vi "DictVectorizer.vi"(8 "error in":errorcluster caption="entrée d'erreur", 11 "DictVectorizer":T1={"dtype"="float", "separator"="=", "sparse"=TRUE, "sort"=TRUE}) -> (0 "error out":errorcluster caption="sortie d'erreur", 3 "DictVectorizer.lvclass":refnum<class "DictVectorizer.lvclass">)   [LabVIEW 2020]
doc: "Transforms lists of feature-value mappings to vectors.\n\nThis transformer turns lists of mappings (dict-like objects) of feature names to feature values into Numpy arrays or scipy.sparse matrices for use with scikit-learn estimators.\n\nWhen feature values are strings, this transformer will do a binary one-hot (aka one-of-K) coding: one boolean-valued feature is constructed for each of the possible string values that the feature can take on. For instance, a feature “f” that can take on the values “ham” and “spam” will become two features in the output, one signifying “f=ham”, the other “f=spam”.\n\nHowever, note that this transformer will only do a binary one-hot encoding when feature values are of type string. If categorical features are represented as numeric values such as int, the DictVectorizer can be followed by sklearn.preprocessing.OneHotEncoder to complete binary one-hot encoding.\n\nFeatures that do not occur in a sample (mapping) will have a zero value in the resulting array/matrix.\n\n\nParameters : \n\n- dtyped : type, default=np.float64\nThe type of feature values. Passed to Numpy array/scipy.sparse matrix constructors as the dtype argument.\n\n- separator : str, default=”=”\nSeparator string used when constructing new features for one-hot coding.\n\n- sparse : bool, default=True\nWhether transform should produce scipy.sparse matrices.\n\n- sort : bool, default=True\nWhether feature_names_ and vocabulary_ should be sorted when fitting.\n\n\nMethods : \n\n- Fit : Learn a list of feature name -> indices mappings.\n\nParameters : X : Mapping or iterable over Mappings\n Dict(s) or Mapping(s) from feature names (arbitrary Python objects) to feature values (strings or convertible to dtype).\n\n- Fit Transform : Learn a list of feature name -> indices mappings and transform X. Like fit(X) followed by transform(X), but does not require materializing X in memory.\n\nParameters : X : Mapping or iterable over Mappings\n Dict(s) or Mapping(s) from feature names (arbitrary Python objects) to feature values (strings or convertible to dtype).\n\nReturns : Xa : {array, sparse matrix}\n Feature vectors; always 2-d.\n \n- Get Feature Names : Returns a list of feature names, ordered by their indices. If one-of-K coding is applied to categorical features, this will include the constructed feature names but not the original ones.\n\n\n- Transform : Transform feature->value dicts to array or sparse matrix. Named features not encountered during fit or fit_transform will be silently ignored.\n\nParameters : X : Mapping or iterable over Mappings of shape (n_samples,)\n Dict(s) or Mapping(s) from feature names (arbitrary Python objects) to feature values (strings or convertible to dtype).\n\nReturns : Xa : {array, sparse matrix}\n Feature vectors; always 2-d."
uses:
  DictVectorizer.lvclass
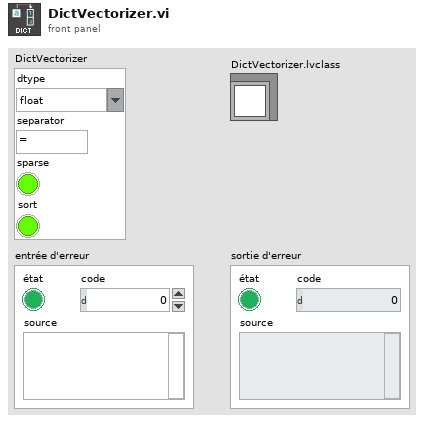
[diagram p1: front panel]
types:
  T1 = cluster{"dtype":string, "separator":string, "sparse":bool, "sort":bool}
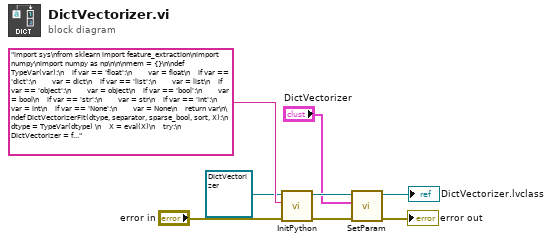
[diagram p0: block diagram]
diagram:
  n1 = call-dynamic "InitPython.vi"("error in (no error)"="error in", "Python Instruction"="import sys\nfrom sklearn import feature_extraction\nimport numpy\nimport numpy as np\n\n\nmem = {}\n\ndef TypeVar(var):\n    if var == 'float':\n        var = float\n    if var == 'dict':\n        var = dict\n    if var == 'list':\n        var = list\n    if var == 'object':\n        var = object\n    if var == 'bool':\n        var = bool\n    if var == 'str':\n        var = str\n    if var == 'int':\n        var = int\n    if var == 'None':\n        var = None\n    return var\n\ndef DictVectorizerFit(dtype, separator, sparse_bool, sort, X):\n    dtype = TypeVar(dtype) \n    X = eval(X)\n    try:\n        DictVectorizer = feature_extraction.DictVectorizer(dtype, separator, sparse_bool, sort).fit(X)\n        mem['FitDictVectorizer'] = DictVectorizer\n        return str('OK')\n    except:\n        erreur = sys.exc_info()\n        typerr = u\"%s\" % (erreur[0])\n        typerr = typerr[typerr.find(\"'\")+1:typerr.rfind(\"'\")]\n        msgerr = u\"%s\" % (erreur[1])\n        message = str('/!\\\\ {0} : {1}'. format(typerr,msgerr))\n        return message \n\ndef DictVectorizerFitTransform(dtype, separator, sparse_bool, sort, X):\n    dtype = TypeVar(dtype)   \n    X = eval(X)\n    try:\n        DictVectorizer = feature_extraction.DictVectorizer(dtype, separator, sparse_bool, sort).fit_transform(X)\n        dtype = type(DictVectorizer)\n        if dtype == numpy.ndarray:\n            DictVectorizer = DictVectorizer.tolist()\n            return str(DictVectorizer)\n        else:\n            Mat = DictVectorizer.tocoo()\n            return str(list(zip(Mat.row, Mat.col, Mat.data)))\n    except:\n        erreur = sys.exc_info()\n        typerr = u\"%s\" % (erreur[0])\n        typerr = typerr[typerr.find(\"'\")+1:typerr.rfind(\"'\")]\n        msgerr = u\"%s\" % (erreur[1])\n        message = str('/!\\\\ {0} : {1}'. format(typerr,msgerr))\n        return message \n    \ndef DictVectorizerGetFeatureNames(dtype, separator, sparse_bool, sort, X):\n    dtype = TypeVar(dtype)    \n    try:\n        DictVectorizer = feature_extraction.DictVectorizer(dtype, separator, sparse_bool, sort).get_feature_names()\n        return str(DictVectorizer)\n    except:\n        erreur = sys.exc_info()\n        typerr = u\"%s\" % (erreur[0])\n        typerr = typerr[typerr.find(\"'\")+1:typerr.rfind(\"'\")]\n        msgerr = u\"%s\" % (erreur[1])\n        message = str('/!\\\\ {0} : {1}'. format(typerr,msgerr))\n        return message \n\ndef DictVectorizerTransform(dtype, separator, sparse_bool, sort, X):\n    dtype = TypeVar(dtype)    \n    X = eval(X)\n    try:\n        DictVectorizerTransform = mem['FitDictVectorizer'].transform(X)\n        dtype = type(DictVectorizerTransform)\n        if dtype == numpy.ndarray:\n            DictVectorizerTransform = DictVectorizerTransform.tolist()\n            return str(DictVectorizerTransform)\n        else:\n            Mat = DictVectorizerTransform.tocoo()\n            return str(list(zip(Mat.row, Mat.col, Mat.data)))\n    except:\n        erreur = sys.exc_info()\n        typerr = u\"%s\" % (erreur[0])\n        typerr = typerr[typerr.find(\"'\")+1:typerr.rfind(\"'\")]\n        msgerr = u\"%s\" % (erreur[1])\n        message = str('/!\\\\ {0} : {1}'. format(typerr,msgerr))\n        return message", "Scikit-learn en entrée"=refnum<class "DictVectorizer.lvclass"> refnum ("DictVectorizer.lvclass")) -> ("error out"=w4:errorcluster, "Scikit-learn en sortie"=w5:refnum<class "DictVectorizer.lvclass">)  [unwired: 7 in]
  n2 = call-dynamic "SetParam.vi"("error in (no error)"=w4, "DictVectorizer"="DictVectorizer", "DictVectorizer.lvclass"=w5) -> ("error out"=→"error out":errorcluster, "DictVectorizer.lvclass"=→"DictVectorizer.lvclass":refnum<class "DictVectorizer.lvclass">)  [unwired: 7 in]
